vi "Write TDATA Core.vi"(10 "raw data":bool[](array[boolean]), 11 "niInstr AXI4-Stream Writer FXP64x4 v1 FPGA in":refnum<class "niInstr AXI4-Stream Writer FXP64x4 v1 FPGA.lvclass">) -> (3 "niInstr AXI4-Stream Writer FXP64x4 v1 FPGA out":refnum<class "niInstr AXI4-Stream Writer FXP64x4 v1 FPGA.lvclass">)   [LabVIEW 2015, in "niInstr AXI4-Stream Writer FXP64x4 v1 FPGA.lvclass"]
uses:
  <instrlib>/_niInstr/CLIP Adapters/v1/FPGA/AXI4-Stream/Writer FXP64x4/niInstr AXI4-Stream Writer FXP64x4 v1 FPGA.lvclass
  <instrlib>/_niInstr/CLIP Adapters/v1/FPGA/AXI4-Stream/Writer FXP64x4/niInstr AXI4-Stream Writer FXP64x4 v1 FPGA.lvclass/niInstr AXI4-Stream Writer FXP64x4 v1 FPGA.ctl
  <vilib>/rvi/eio/common/nirviEmuTemplateMethod_errors.vi
  <instrlib>/_niInstr/Data Formatting/v1/FPGA/Private/Convert/Boolean Array to U64 Array.vi
  <vilib>/eio/EIONode/EIONode.xnode
  <instrlib>/_niInstr/Data Formatting/v1/FPGA/niInstr Data Formatting v1 FPGA.lvlib
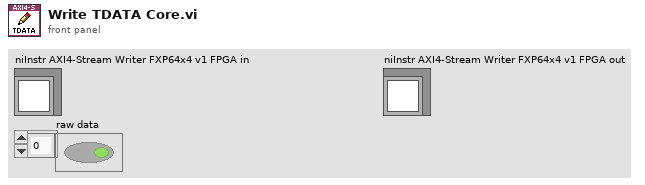
[diagram p1: front panel]
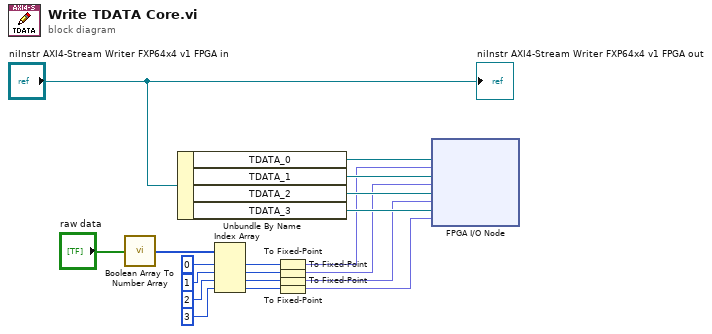
[diagram p0: block diagram]
diagram:
  n1 = call-poly <instrlib>:"Boolean Array To Number Array.vi"("data in"="raw data") -> ("data out"=w9:u64[])  [unwired: 14 in]
  n2 = Unbundle By Name("niInstr AXI4-Stream Writer FXP64x4 v1 FPGA in") -> ("TDATA_0"=w19:refnum<k21>, "TDATA_1"=w18:refnum<k21>, "TDATA_2"=w13:refnum<k21>, "TDATA_3"=w12:refnum<k21>)
  n3 = Index Array(array=w9, index #1=0 ("index"), index #2=1 ("index"), index #3=2 ("index"), index #4=3 ("index")) -> (element #1=w8:u64, element #2=w7:u64, element #3=w6:u64, element #4=w5:u64)
  n4 = To Fixed-Point(number=w8) -> (fixed-point=w4:fxp<+,64,64>)  [unwired: 1 in]
  n5 = To Fixed-Point(number=w7) -> (fixed-point=w3:fxp<+,64,64>)  [unwired: 1 in]
  n6 = To Fixed-Point(number=w6) -> (fixed-point=w2:fxp<+,64,64>)  [unwired: 1 in]
  n7 = To Fixed-Point(number=w5) -> (fixed-point=w1:fxp<+,64,64>)  [unwired: 1 in]
  n8 = xnode "FPGA I/O Node"("I/O Item"=w4, "FPGA I/O In"=w19, "I/O Item"=w3, "FPGA I/O In"=w18, "I/O Item"=w2, "FPGA I/O In"=w13, "I/O Item"=w1, "FPGA I/O In"=w12) -> ()  [unwired: 4 out]
  "niInstr AXI4-Stream Writer FXP64x4 v1 FPGA out" <- "niInstr AXI4-Stream Writer FXP64x4 v1 FPGA in"
